vi "serial_get.vi"(5 "command":string, 7 "serial_send":bool, 8 "error in (no error)":errorcluster, 9 "serial_connected_in":bool, 10 "new_connection":bool, 11 "VISA_refnum_in":refnum<visa-resource-name>) -> (0 "error out":errorcluster, 1 "serial_connected_out":bool, 3 "VISA_Refnum_out":refnum<visa-resource-name>, 4 "read_buffer_out":string, 6 "new_data_available":bool)   [LabVIEW 2025]
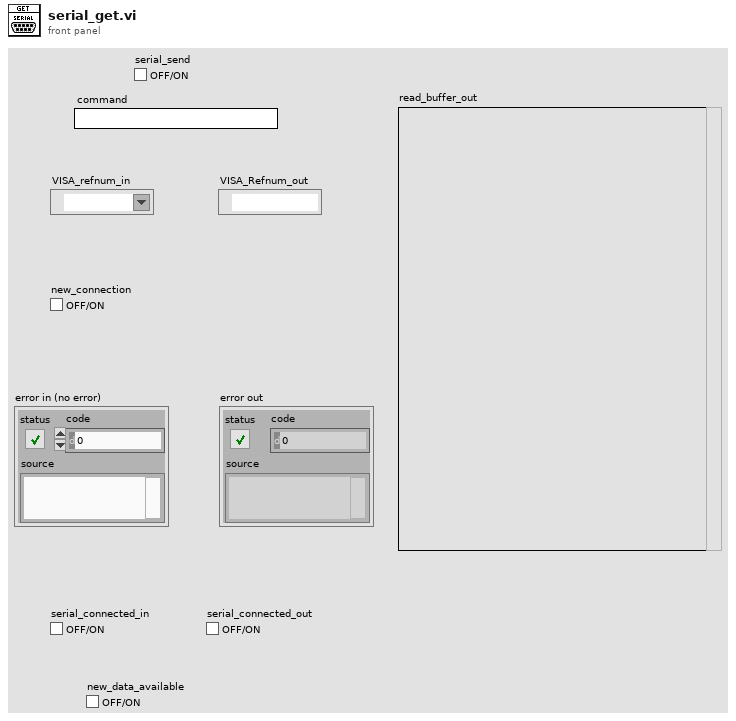
[diagram p1: front panel]
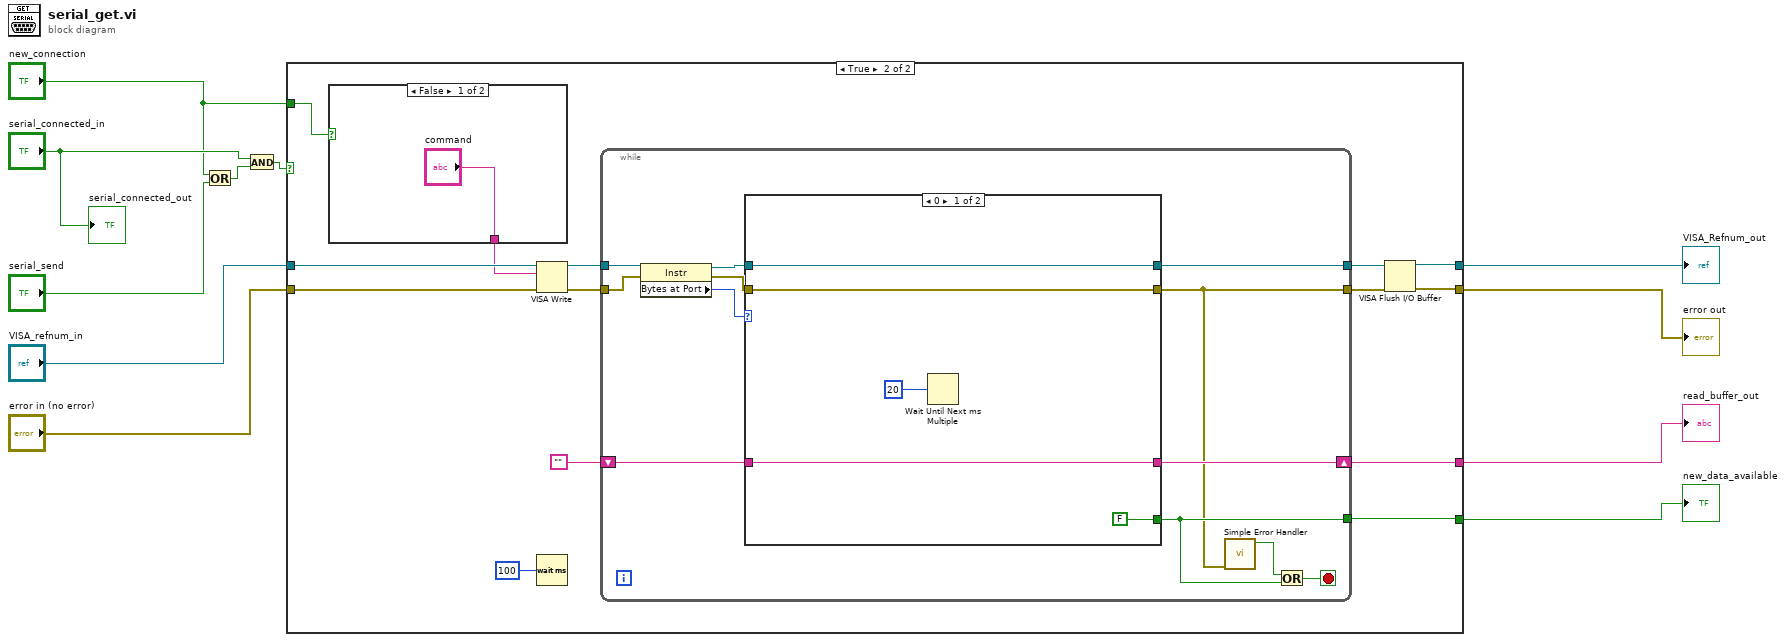
[diagram p0: block diagram]
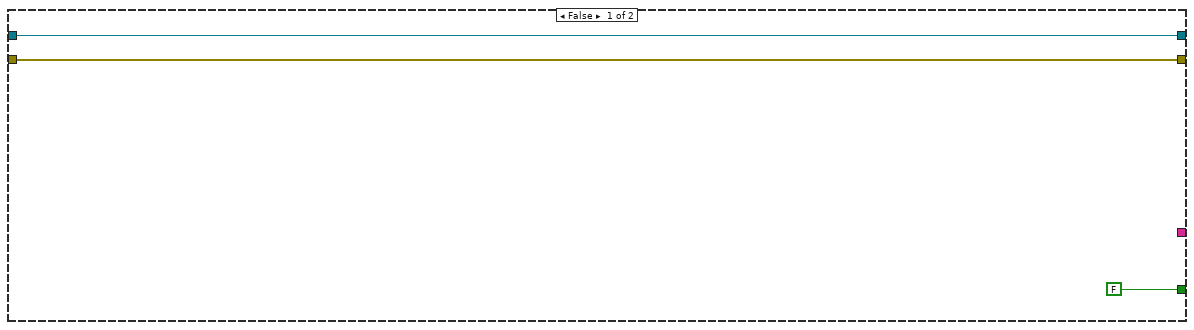
[diagram p2: hidden frame]
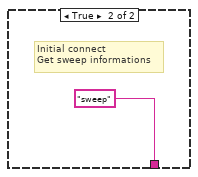
[diagram p3: hidden frame]
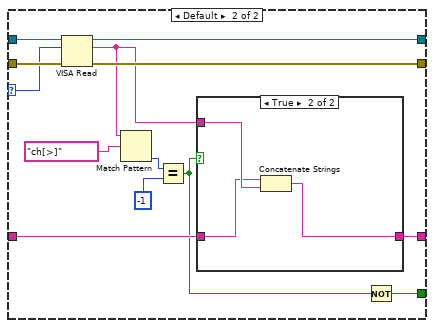
[diagram p4: hidden frame]
diagram:
  n1 = Or(x="new_connection", y="serial_send") -> (x .or. y?=w3:bool)
  n2 = And(x="serial_connected_in", y=w3) -> (x .and. y?=w6:bool)
  n3 = case shown="True" w6 {
    tunnel: [_ w28] -> w8
    tunnel: [FALSE w27] -> w9
    tunnel: "VISA_refnum_in" -> [w14 w26]
    tunnel: "error in (no error)" -> [w13 w25]
    tunnel: [w13 w15] -> w5
    tunnel: [w14 w17] -> w11
    tunnel: "new_connection" -> [_ w20]
    frame False {
    }
    frame True {
      n4 = case shown="False" w20 {
        tunnel: ["command" "sweep"] -> w19
        frame False {
        }
        frame True {
          # "Initial connect\nGet sweep informations"
        }
      }
      n5 = VISA Write(VISA resource name=w26, write buffer=w19, error in (no error)=w25) -> (VISA resource name out=w23:refnum<visa-resource-name>, error out=w24:errorcluster)  [unwired: 1 out]
      n6 = Wait (ms)(milliseconds to wait=u32 100) -> ()  [unwired: 1 out]
      n7 = while {
        shift-right: [w41] -> w28
        shift-left: "" -> [w42]
        tunnel: w23 -> [w37]
        tunnel: w24 -> [w38]
        tunnel: [w31] -> w16
        tunnel: [w34] -> w27
        tunnel: [w32] -> w18
        stop <- w35 stop-if-true
        n8 = property class="Instr"(reference=w37, error in=w38) -> (reference out=w40:refnum<visa-resource-name>, error out=w39:errorcluster, "Bytes at Port"=w36:u32)
        n9 = case shown="0" w36 {
          selector: w36 -> [_ w54]
          tunnel: w40 -> [w47 w57]
          tunnel: w39 -> [w46 w58]
          tunnel: [w47 w60] -> w32
          tunnel: [w46 w59] -> w31
          tunnel: w42 -> [w44 w55]
          tunnel: [w44 w56] -> w41
          tunnel: [FALSE w49] -> w34
          frame 0 {
            n10 = Wait Until Next ms Multiple(millisecond multiple=u32 20) -> ()  [unwired: 1 out]
          }
          frame Default {
            n11 = VISA Read(VISA resource name=w57, byte count=w54, error in (no error)=w58) -> (VISA resource name out=w60:refnum<visa-resource-name>, read buffer=w51:string, error out=w59:errorcluster)  [unwired: 1 out]
            n12 = Match Pattern(string=w51, regular expression="ch[>]" ("y")) -> (offset past match=w53:i32)  [unwired: 1 in, 3 out]
            n13 = Equal?(x=w53, y=-1) -> (x = y?=w48:bool)
            n14 = case shown="True" w48 {
              tunnel: [w61 w64] -> w56
              tunnel: w51 -> [_ w63]
              tunnel: w55 -> [w61 w62]
              frame False {
              }
              frame True {
                n15 = Concatenate Strings(w62, w63) -> (w64:string)
              }
            }
            n16 = Not(x=w48) -> (.not. x?=w49:bool)
          }
        }
        n17 = call <vilib>:"Simple Error Handler.vi"("error in (no error)"=w31) -> ("error?"=w33:bool)  [unwired: 4 in, 4 out]
        n18 = Or(x=w33, y=w34) -> (x .or. y?=w35:bool)
      }
      n19 = VISA Flush I/O Buffer(VISA resource name=w18, error in (no error)=w16) -> (VISA resource name out=w17:refnum<visa-resource-name>, error out=w15:errorcluster)  [unwired: 1 in]
    }
  }
  "error out" <- w5
  "VISA_Refnum_out" <- w11
  "new_data_available" <- w9
  "read_buffer_out" <- w8
  "serial_connected_out" <- "serial_connected_in"
